vi "Main (1).vi"() -> ()   [LabVIEW 2013]
uses:
  <vilib>/myRIO/Common/Instrument Driver Framework/myRIO v1.0/UART/vis/myRIO v1.0 Close UART.vi
  <vilib>/functionblocks/Edge Detection/One Shot Rising with Input/One Shot Rising with Input.vi
  <vilib>/myRIO/Common/Instrument Driver Framework/Utilities/vis/FPGA Ref Manager.vi
  <vilib>/myRIO/Common/Instrument Driver Framework/myRIO v1.0/myRIO v1.0 Reset FPGA.vi
  <vilib>/functionblocks/FB Core/FB Core.xnode
  <vilib>/myRIO/Instrument Drivers/Utilities/Utilities.lvlib
  <vilib>/functionblocks/NI_FunctionBlock Libraries.lvlib
panel:
  in  "Tab Control 2":T1(tab)
  in  "Y Accel Rate (mm/s^2)":dbl
  in  "Y Decel Rate (mm/s^2)":dbl
  in  "Y Vmax (mm/s)":dbl
  in  "Y Vcreep (mm/s)":dbl
  in  "Y Creep  Distance (mm)":dbl
  in  "Y Overrun Distance (mm)":dbl
  in  "Y Target Coordinate Override (mm)":dbl min=0.0
  in  "Enable Y Coordinate Override":bool
  in  "Y-Axis Direction Request":bool
  in  "Y Axis Speed Override (mm/s)":dbl format="%#_13g"
  in  "Enable Y Axis Override":bool
  in  "Tab Control":T2(tab)
  in  "X Vmax (mm/s)":dbl
  in  "X Vcreep (mm/s)":dbl
  in  "X Overrun Distance (mm)":dbl
  in  "X Decel Rate (mm/s^2)":dbl
  in  "X Creep  Distance (mm)":dbl
  in  "X Accel Rate (mm/s^2)":dbl
  in  "X Target Coordinate (mm) 2":dbl min=0.0
  in  "Enable X Coordinate Override":bool
  in  "Enable X Axis Override":bool
  in  "X Axis Speed Override (mm/s)":dbl format="%#_13g"
  in  "X-Axis Direction Request":bool
  out "X Movement Timeout (s)":dbl caption="Elapsed Time (s)"
  out "X Target Coordinate (mm)":dbl min=0.0
  out "Y Target Coordinate (mm)":dbl min=0.0
  in  "Move to Specified Coordinate":bool
  in  "Calibrate Axes":bool
  out "Y Axis Frequency Command":dbl
  out "Y Axis Direction Command 3":bool
  out "Y_FiltSpeed(mm/s)":dbl
  out "Y_Dist_mm@(N)":dbl
  out "Y Axis":cluster{"Y":dbl[], "Y":dbl[]}[](graph)
  out "Y Speed Command (mm/s)":dbl
  out "Y Selected Speed Control Case":T3(ring)
  out "Active Y Axis Control Case":T4(ring)
  out "Active X Axis Control Case":T4(ring)
  out "X Speed Command (mm/s)":dbl
  out "X Selected Speed Control Case":T3(ring)
  out "X Axis":cluster{"Y":dbl[], "Y":dbl[]}[](graph)
  out "X_Dist_mm@(N)":dbl
  out "X_FiltSpeed(mm/s)":dbl
  out "X Axis Direction Command":bool
  out "X Axis Duty Command":dbl
  in  "Stop Button":bool
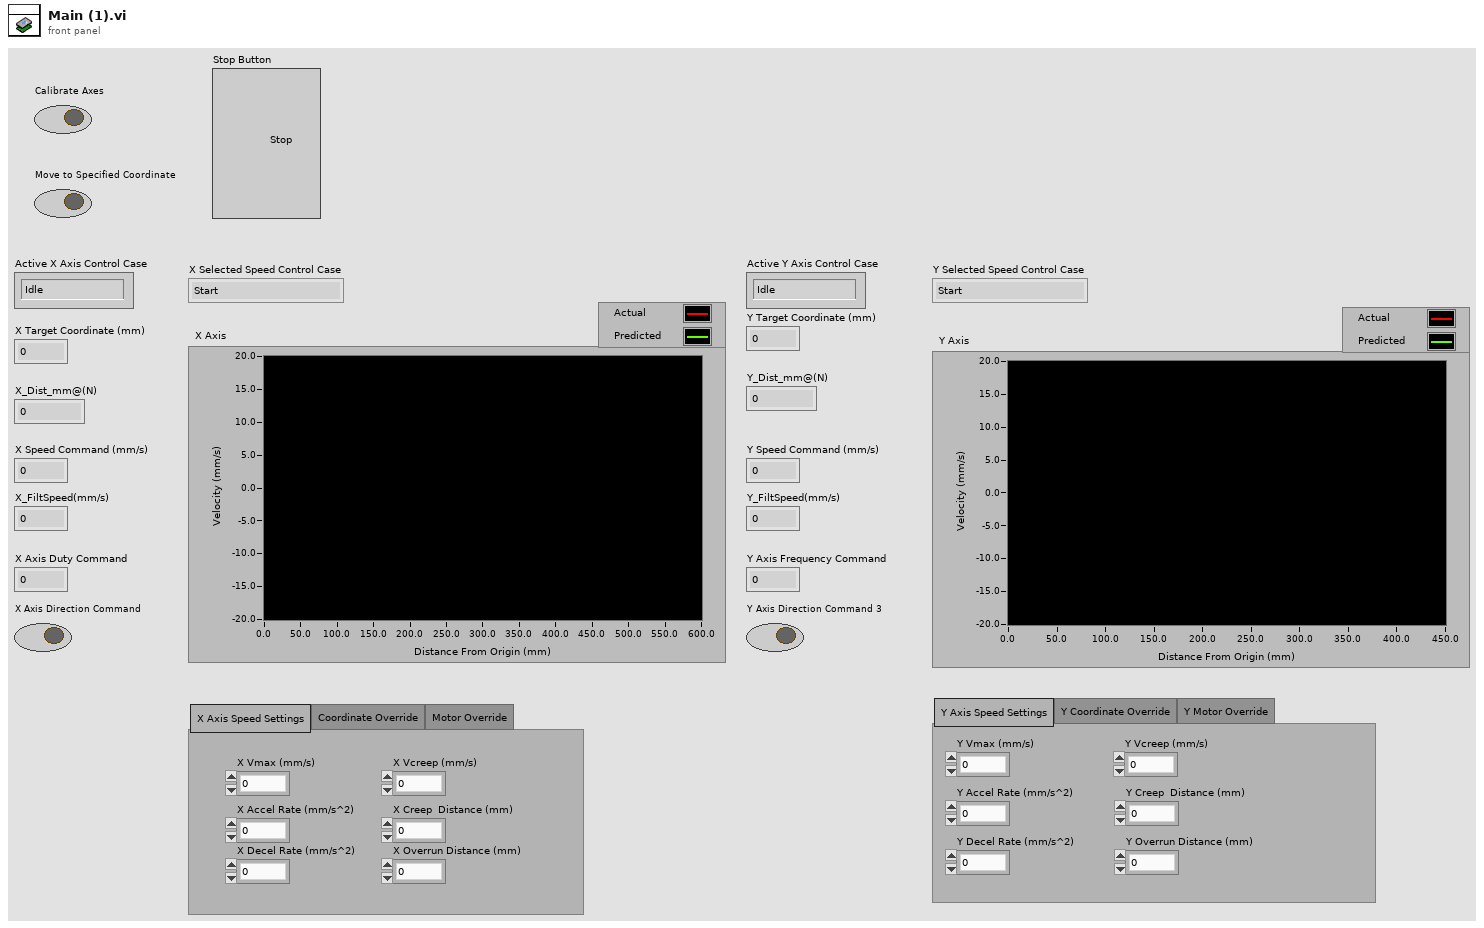
[diagram p1: front panel]
types:
  T1 = enum32{"Y Axis Speed Settings", "Y Coordinate Override", "Y Motor Override"}
  T2 = enum32{"X Axis Speed Settings", "Coordinate Override", "Motor Override"}
  T3 = enum16{"Start", "Accelerate", "Hold Vmax", "Decelerate", "Hold at Vcreep", "Stop"}
  T4 = enum16{"Idle", "PredictProfile", "Calibrate", "Home", "Go to Coordinate"}
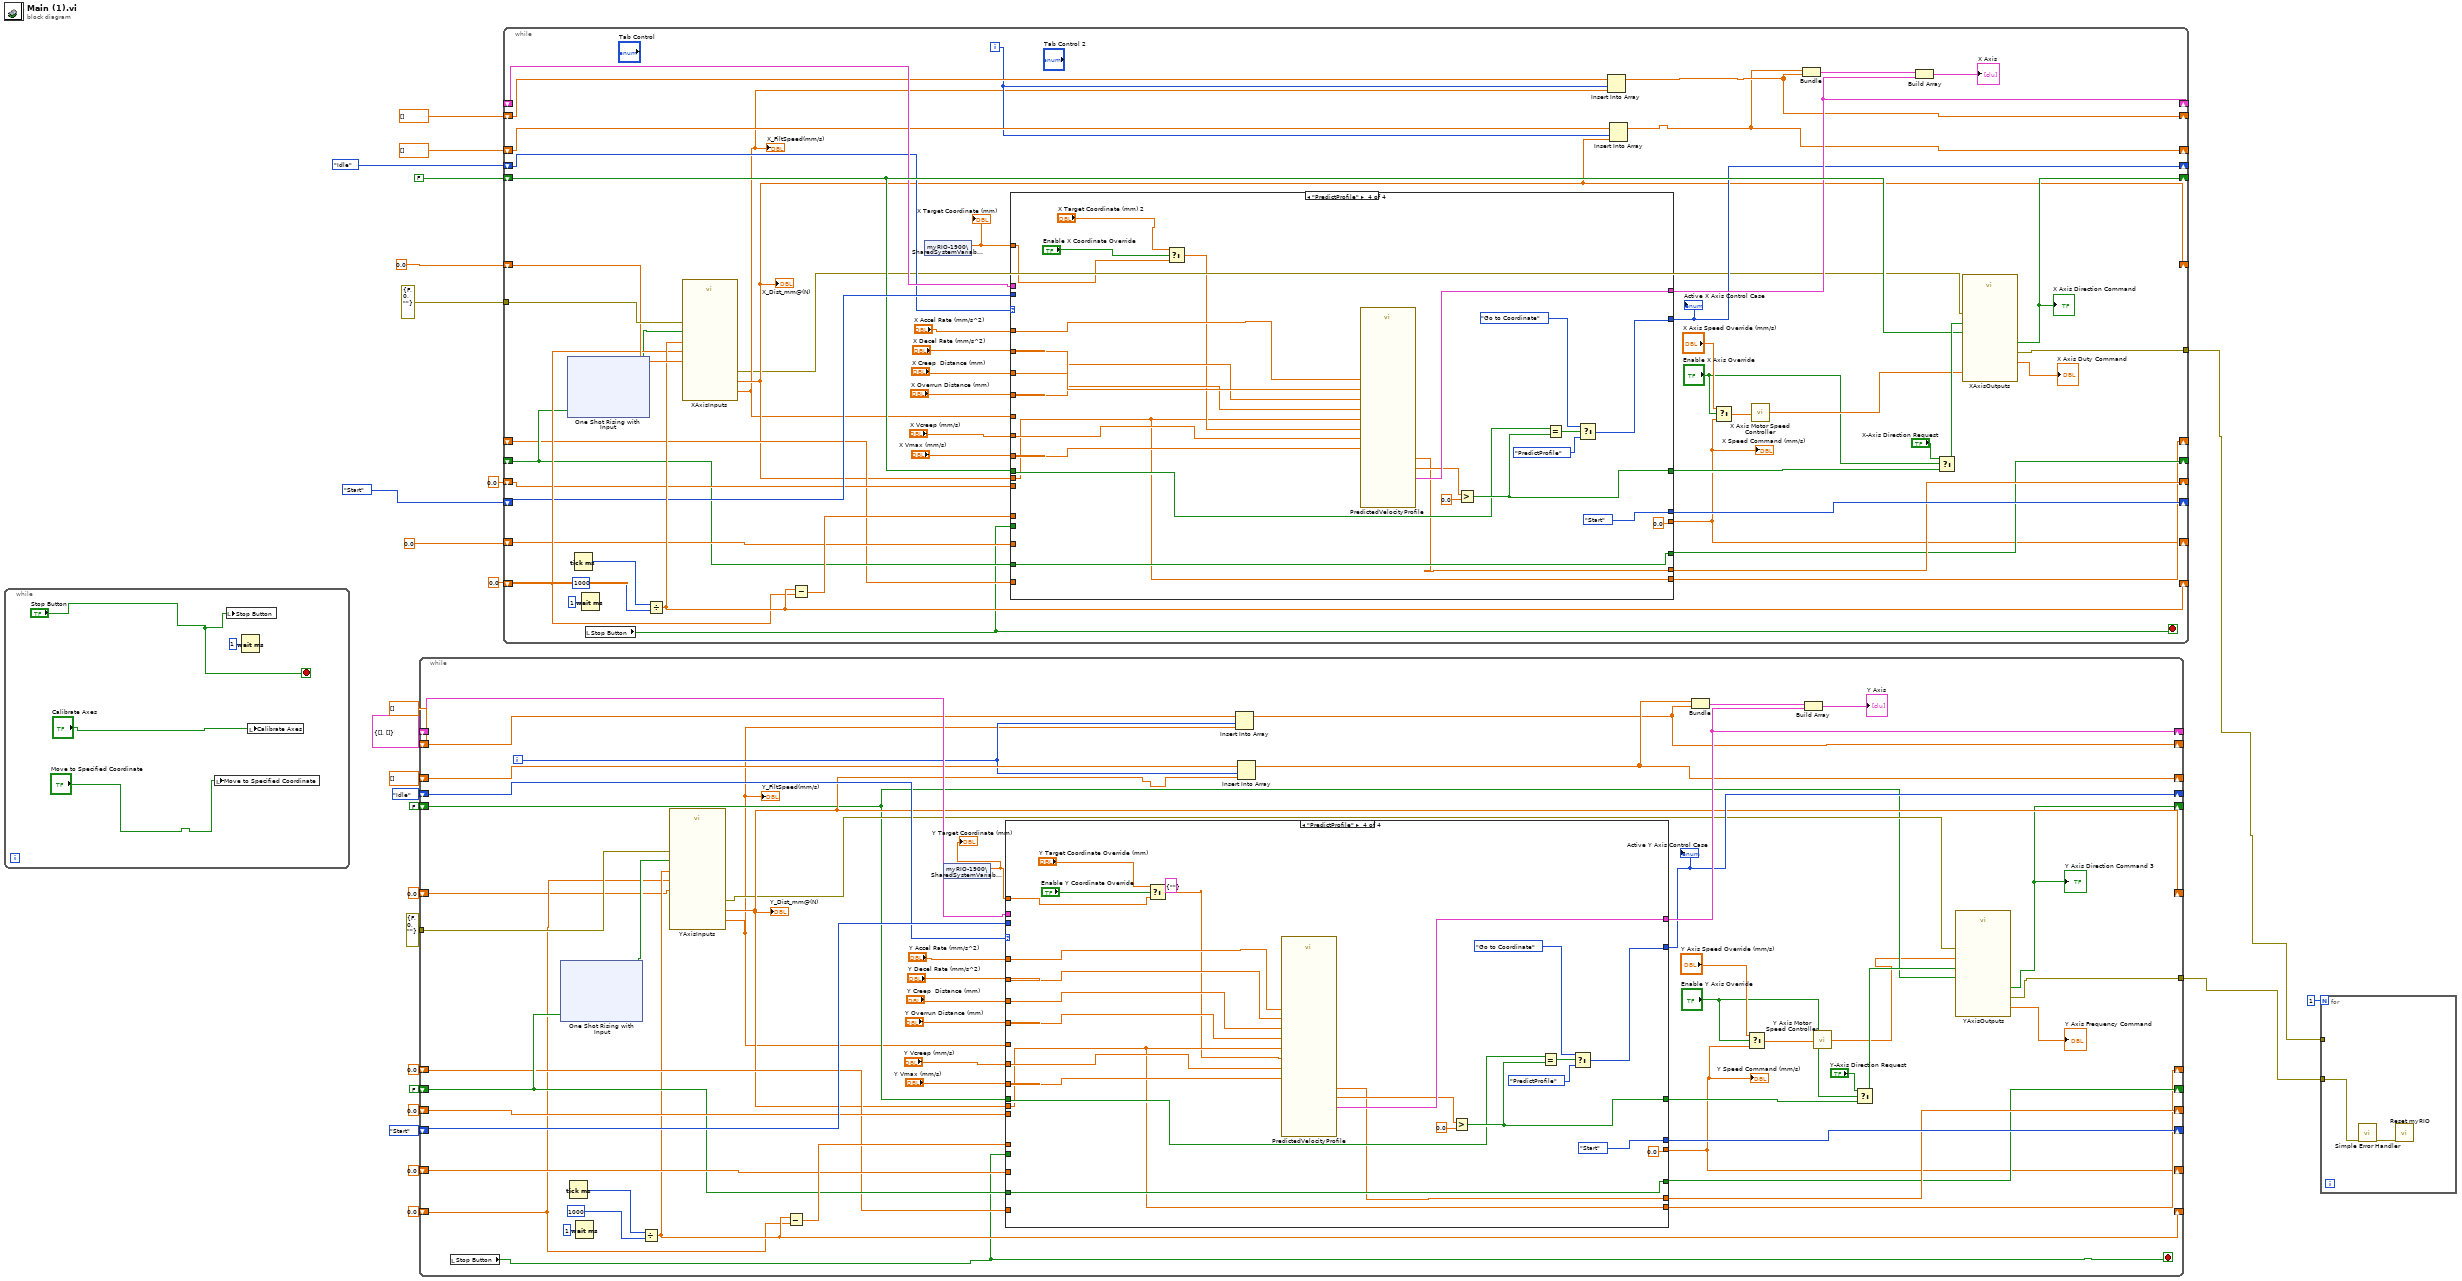
[diagram p0: block diagram]
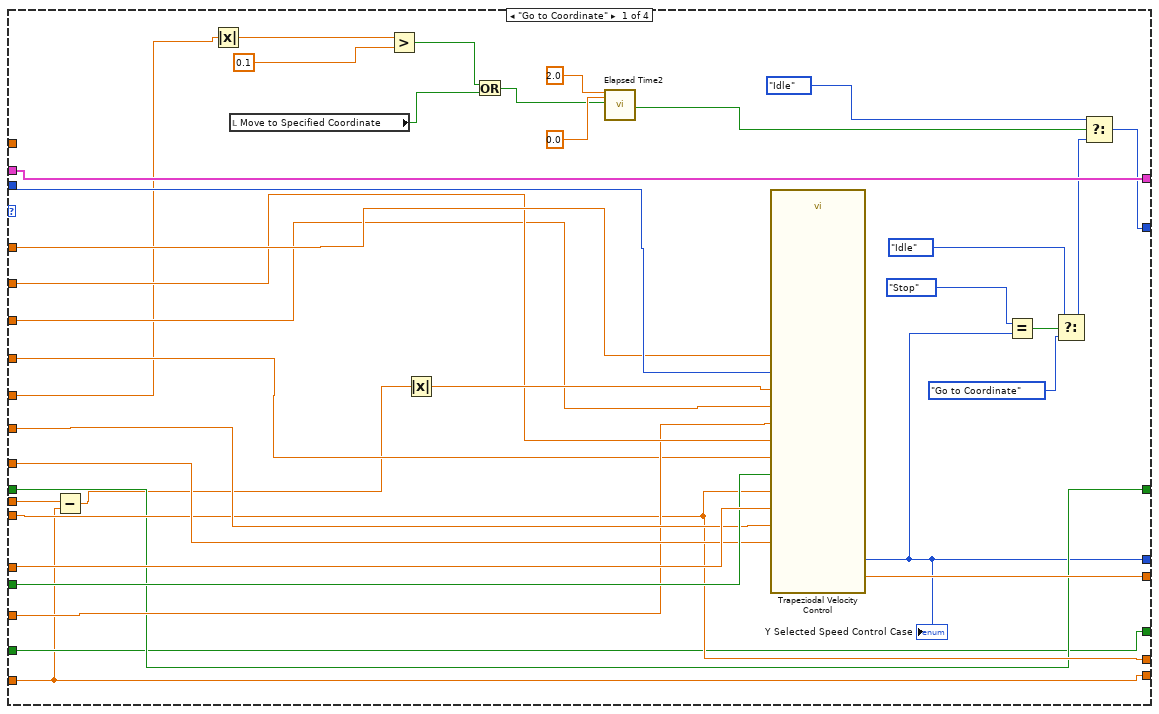
[diagram p2: hidden frame]
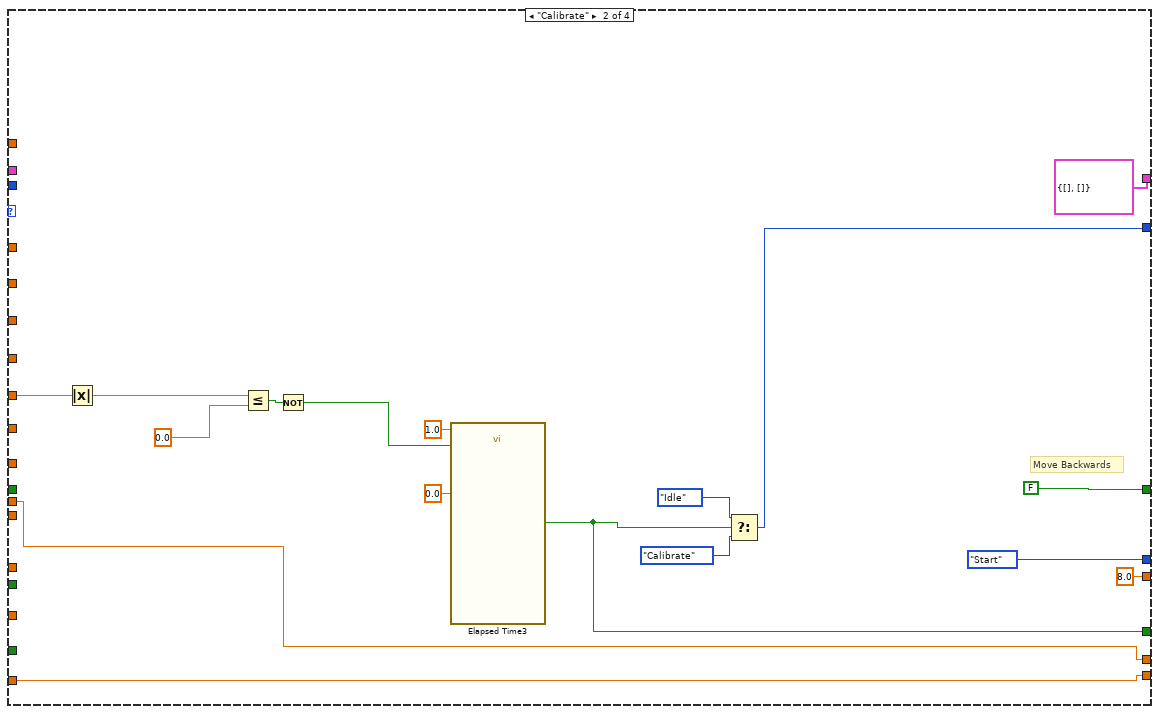
[diagram p3: hidden frame]
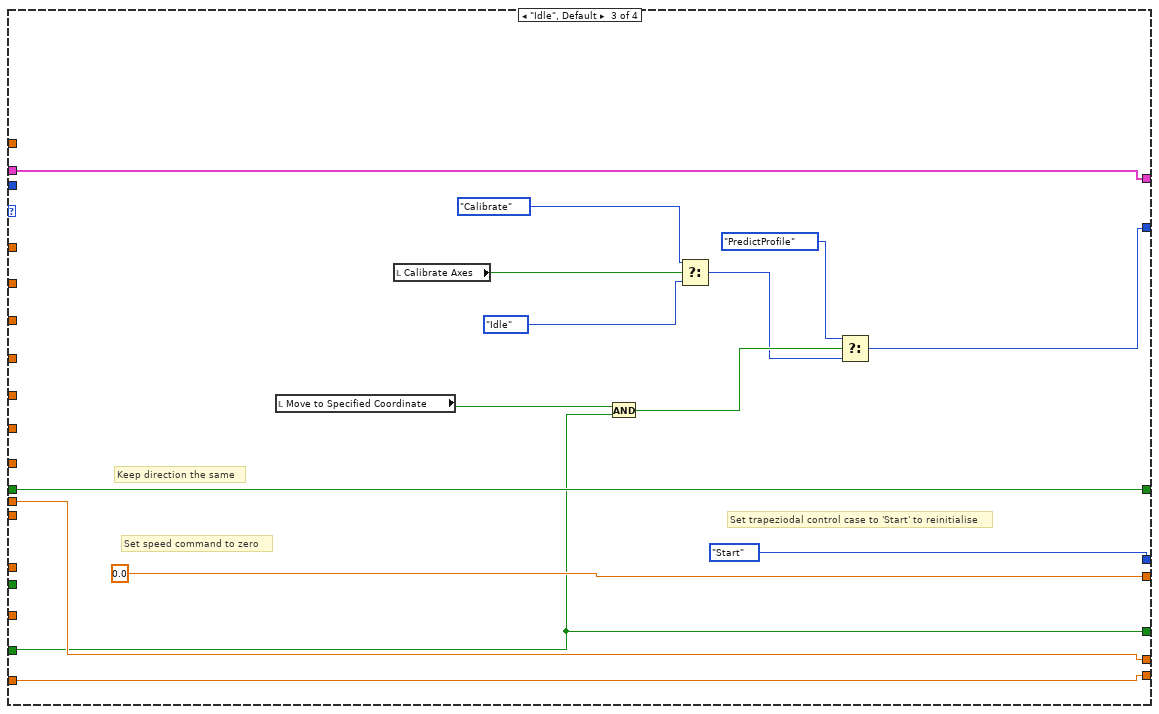
[diagram p4: hidden frame]
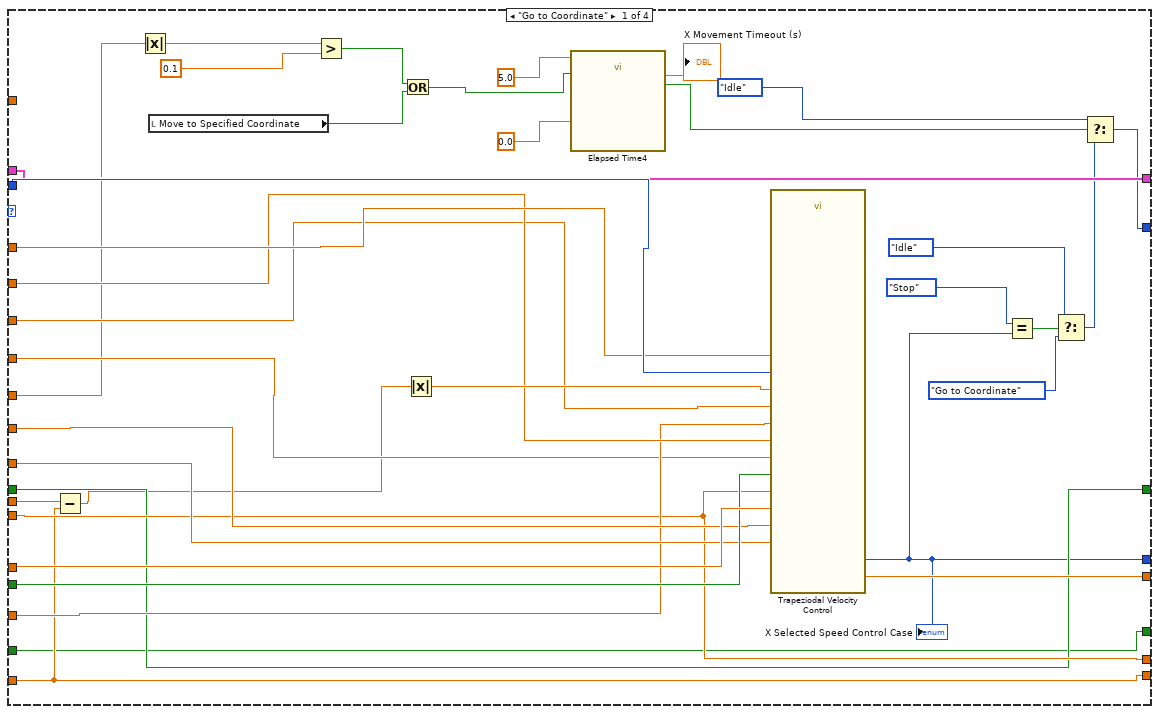
[diagram p5: hidden frame]
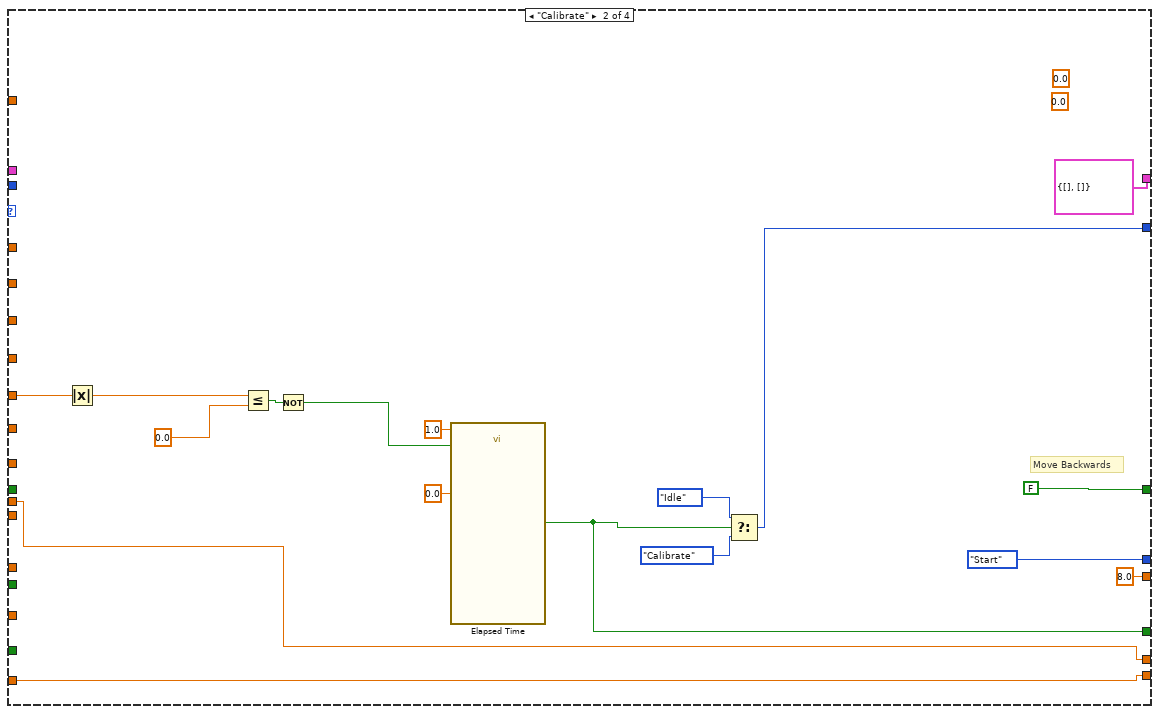
[diagram p6: hidden frame]
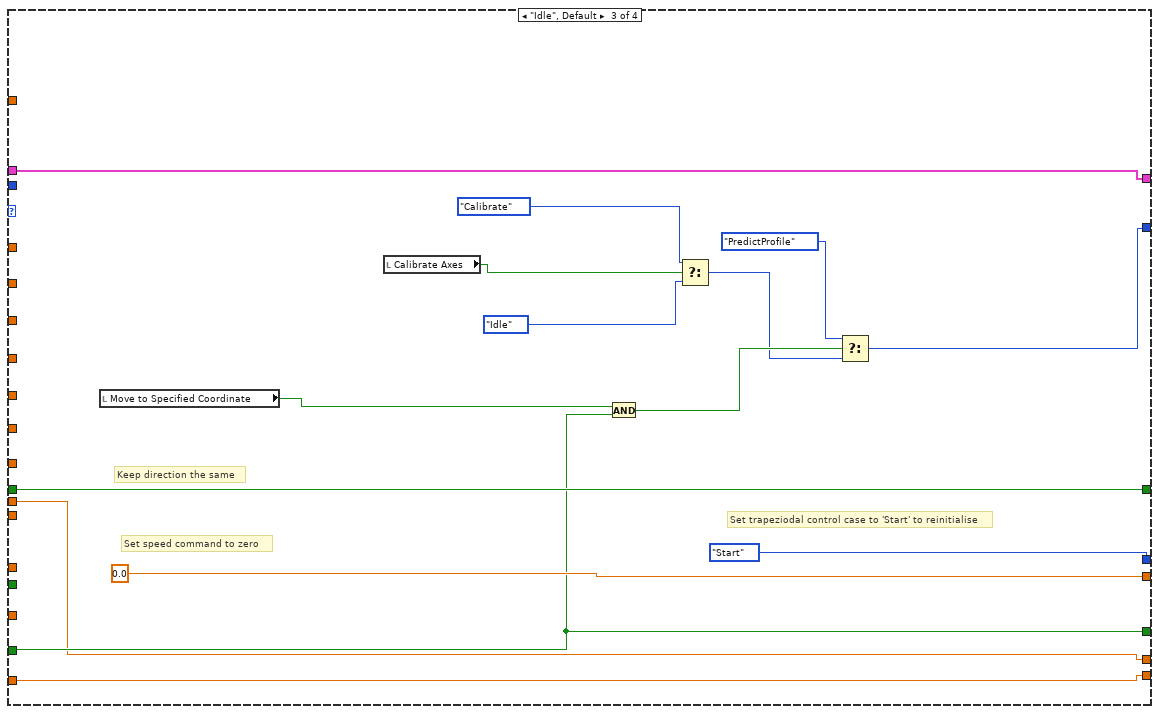
[diagram p7: hidden frame]
diagram:
  n1 = while {
    stop <- "Stop Button" stop-if-true
    n2 = local write "Move to Specified Coordinate"("Move to Specified Coordinate") -> ()
    n3 = local write "Stop Button"("Stop Button") -> ()
    n4 = Wait (ms)(milliseconds to wait=u32 1) -> ()  [unwired: 1 out]
    n5 = local write "Calibrate Axes"("Calibrate Axes") -> ()
  }
  n6 = while {
    shift-right: [w48] -> _
    shift-left: 0.0 -> [w46]
    tunnel: errorcluster {"status"=FALSE, "code"=0, "source"=""} ("error in (no error)") -> [w50]
    shift-right: [w41] -> _
    shift-left: FALSE ("Direction Command") -> [w42]
    tunnel: [w40] -> w1
    shift-right: [w47] -> _
    shift-left: 0.0 ("X_Dist_mm@(N)") -> [w45]
    shift-right: [w79] -> _
    shift-left: T3."Start" ("Selected Speed Control Case") -> [w74]
    shift-right: [w35] -> _
    shift-left: 0.0 ("Speed Command (mm/s)") -> [w66]
    shift-right: [w59] -> _
    shift-left: dbl[] [] -> [w57]
    shift-right: [w58] -> _
    shift-left: dbl[] [] -> [w54]
    shift-right: [w65] -> _
    shift-left: 0.0 ("Absolute Distance to Move (mm)") -> [w64]
    shift-right: [w63] -> _
    shift-left: cluster{dbl[], cdb[]} {[], []} ("PredictedVelocityProfile") -> [w62]
    shift-right: [w61] -> _
    shift-left: T4."Idle" ("Active X Axis Control Case") -> [w53]
    shift-right: [w60] -> _
    shift-left: FALSE ("Time has Elapsed") -> [w56]
    shift-right: [w52] -> _
    shift-left: 0.0 ("X_Dist_mm@(N)") -> [w51]
    i -> [w55]
    stop <- w32 stop-if-true
    n7 = local read "Stop Button"() -> (w32:bool)
    n8 = xnode "One Shot Rising with Input"("input"=w56) -> ("output"=w49:bool)  [unwired: 1 in, 1 out]
    n9 = Tick Count (ms)() -> (millisecond timer value=w81:u32)
    n10 = Wait (ms)(milliseconds to wait=u32 1) -> ()  [unwired: 1 out]
    n11 = Divide(x=w81, y=u32 1000) -> (x/y=w48:dbl)
    n12 = call "YAxisInputs.vi"("t_s"=w48, "error in (no error)"=w50, "t_s@(N-1)"=w46, "Reset Timer and Encoder Counts"=w49, "Y_Dist_mm@(N-1)"=w45) -> ("error out"=w44:errorcluster, "Y_Dist_mm@(N)"=w47:dbl, "Y_FiltSpeed(mm/s)"=w34:dbl)  [unwired: 4 in]
    "Y_FiltSpeed(mm/s)" <- w34
    "Y_Dist_mm@(N)" <- w47
    n13 = Subtract(x=w48, y=w46) -> (x-y=w78:dbl)
    n14 = shared-variable "myRIO-1900\\SharedSystemVariables.lvlib\\Puck Y"() -> (w39:dbl)  [unwired: 1 in, 1 out]
    "Y Target Coordinate (mm)" <- w39
    n15 = case shown="\"PredictProfile\"" w53 {
      tunnel: [w141 T3."Start" ("Selected Speed Control Case") T3."Start" ("Selected Speed Control Case") T3."Start" ("Selected Speed Control Case")] -> w79
      tunnel: w78 -> [w156 _ _ _]
      tunnel: w32 -> [w154 _ _ _]
      tunnel: [w153 8.0 ("Speed Command (mm/s)") 0.0 ("Speed Command (mm/s)") 0.0 ("Speed Command (mm/s)")] -> w35
      tunnel: w74 -> [w152 _ _ _]
      tunnel: [w143 FALSE ("Direction Command") w188 w200] -> w73
      tunnel: w42 -> [w143 _ w188 w199]
      tunnel: "Y Accel Rate (mm/s^2)" -> [w151 _ _ w212]
      tunnel: "Y Decel Rate (mm/s^2)" -> [w150 _ _ w211]
      tunnel: "Y Creep  Distance (mm)" -> [w149 _ _ w210]
      tunnel: "Y Overrun Distance (mm)" -> [w145 _ _ w209]
      tunnel: "Y Vcreep (mm/s)" -> [w148 _ _ w208]
      tunnel: "Y Vmax (mm/s)" -> [w147 _ _ w207]
      tunnel: w47 -> [w135 w173 w185 w193]
      tunnel: w66 -> [w146 _ _ _]
      tunnel: [w142 cluster{dbl[], cdb[]} {[], []} ("PredictedVelocityProfile") w178 w206] -> w63
      tunnel: [w144 w173 w185 w194] -> w65
      tunnel: w64 -> [w144 _ _ _]
      tunnel: w62 -> [w142 _ w178 _]
      tunnel: [w127 w166 w176 w196] -> w61
      tunnel: w34 -> [w123 w168 _ _]
      tunnel: [w136 w158 w179 w201] -> w60
      tunnel: w56 -> [w136 _ w179 w201]
      tunnel: [w133 w157 w177 w193] -> w52
      tunnel: w51 -> [w133 w157 w177 _]
      tunnel: w39 -> [_ _ _ w189]
      frame "Go to Coordinate" {
        n16 = Subtract(x=w135, y=w133) -> (x-y=w134:dbl)
        n17 = Absolute Value(x=w123) -> (abs(x)=w125:dbl)
        n18 = local read "Move to Specified Coordinate"() -> (w121:bool)
        n19 = Greater?(x=w125, y=0.1) -> (0:w124:bool)
        n20 = Absolute Value(x=w134) -> (abs(x)=w155:dbl)
        n21 = Or(x=w124, y=w121) -> (x .or. y?=w122:bool)
        n22 = call "Elapsed Time2"("Time Target (s)"=2.0, "Reset"=w122, "Set Start Time (s)"=0.0) -> ("Time has Elapsed"=w129:bool)  [unwired: 9 in, 7 out]
        n23 = call "Trapeziodal Velocity Control.vi"("Active Speed Control Case"=w152, "Vmax (mm/s)"=w147, "Accel Rate (mm/s^2)"=w151, "Decel Rate (mm/s^2) 2"=w150, "Current Speed (mm/s)"=w146, "Target Distance (mm)"=w144, "Actual Distance (mm)"=w155, "Creep  Distance (mm)"=w149, "Vcreep (mm/s)"=w148, "Overrun Distance (mm)"=w145, "Timestep (dt)"=w156, "stop or error"=w154) -> ("Selected Speed Control Case"=w141:T3, "Speed Command (mm/s)"=w153:dbl)  [unwired: 2 in]
        "Y Selected Speed Control Case" <- w141
        n24 = Equal?(x=T3."Stop" ("y"), y=w141) -> (x = y?=w139:bool)
        n25 = Select(t=T4."Idle" ("X Axis Control Case"), s=w139, f=T4."Go to Coordinate" ("X Axis Control Case")) -> (s? t:f=w128:T4)
        n26 = Select(t=T4."Idle" ("X Axis Control Case"), s=w129, f=w128) -> (s? t:f=w127:T4)
      }
      frame "Calibrate" {
        # "Move Backwards"
        n27 = Absolute Value(x=w168) -> (abs(x)=w163:dbl)
        n28 = Less Or Equal?(x=w163, y=0.0) -> (x <= y?=w162:bool)
        n29 = Not(x=w162) -> (.not. x?=w161:bool)
        n30 = call "Elapsed Time3"("Time Target (s)"=1.0, "Reset"=w161, "Set Start Time (s)"=0.0) -> ("Time has Elapsed"=w158:bool)  [unwired: 9 in, 7 out]
        n31 = Select(t=T4."Idle" ("X Axis Control Case"), s=w158, f=T4."Calibrate" ("X Axis Control Case")) -> (s? t:f=w166:T4)
      }
      frame "Idle", Default {
        # "Set trapeziodal control case to 'Start' to reinitialise"
        # "Set speed command to zero"
        # "Keep direction the same"
        n32 = local read "Move to Specified Coordinate"() -> (w174:bool)
        n33 = local read "Calibrate Axes"() -> (w175:bool)
        n34 = And(x=w174, y=w179) -> (x .and. y?=w182:bool)
        n35 = Select(t=T4."Calibrate" ("X Axis Control Case"), s=w175, f=T4."Idle" ("X Axis Control Case")) -> (s? t:f=w181:T4)
        n36 = Select(t=T4."PredictProfile" ("X Axis Control Case"), s=w182, f=w181) -> (s? t:f=w176:T4)
      }
      frame "PredictProfile" {
        (unwired) cluster{"source":string} {"source"=""} ("error in (no error)")
        n37 = Select(t="Y Target Coordinate Override (mm)", s="Enable Y Coordinate Override", f=w189) -> (s? t:f=w190:dbl)
        n38 = call "PredictedVelocityProfile.vi"("Start Coordinate (mm)"=w193, "V_Max_mm/s"=w207, "Accel_mm/s^2"=w212, "Target Coordinate (mm)"=w190, "S_Creep_mm"=w210, "S_Overrun_mm"=w209, "V_Creep_mm/s"=w208, "Decel_mm/s^2"=w211) -> ("Absolute Distance to Move (mm)"=w194:dbl, "Direction Request"=w204:dbl, "PredictedVelocityProfile"=w206:cluster{dbl[], cdb[]})  [unwired: 4 in, 1 out]
        n39 = Greater?(x=w204, y=0.0) -> (0:w200:bool)
        n40 = Equal?(x=w199, y=w200) -> (x = y?=w198:bool)
        n41 = Select(t=T4."Go to Coordinate" ("Active X Axis Control Case"), s=w198, f=T4."PredictProfile" ("Active X Axis Control Case")) -> (s? t:f=w196:T4)
      }
    }
    "Y Speed Command (mm/s)" <- w35
    "Active Y Axis Control Case" <- w61
    n42 = Insert Into Array(array=w54, index=w55, new element=w34) -> (w58:dbl[])
    n43 = Insert Into Array(array=w57, index=w55, new element=w47) -> (w59:dbl[])
    n44 = Bundle(w59, w58) -> (w76:cluster{dbl[], dbl[]})  [unwired: 1 in]
    n45 = Select(t="Y Axis Speed Override (mm/s)", s="Enable Y Axis Override", f=w35) -> (s? t:f=w36:dbl)
    n46 = Build Array(w76, w63) -> (→"Y Axis":cluster{dbl[], cdb[]}[])
    n47 = call "Y Axis Motor Speed Controller.vi"("Speed Command (mm/s)"=w36) -> ("PWM  Frequency Command (Hz)"=w33:dbl)
    n48 = Select(t="Y-Axis Direction Request", s="Enable Y Axis Override", f=w73) -> (s? t:f=w43:bool)
    n49 = call "YAxisOutputs.vi"("error in (no error)"=w44, "PWM  Frequency Command (Hz)"=w33, "YActiveDirectionCmd"=w42, "Y-Axis Direction Request"=w43) -> ("error out"=w40:errorcluster, "Limited Output"=→"Y Axis Frequency Command":dbl, "Direction Command"=w41:bool)  [unwired: 5 in]
    "Y Axis Direction Command 3" <- w41
  }
  n50 = while {
    shift-right: [w255] -> _
    shift-left: 0.0 -> [w254]
    tunnel: errorcluster {"status"=FALSE, "code"=0, "source"=""} ("error in (no error)") -> [w261]
    shift-right: [w259] -> _
    shift-left: FALSE ("Direction Command") -> [w247]
    tunnel: [w258] -> w18
    shift-right: [w224] -> _
    shift-left: 0.0 ("X_Dist_mm@(N)") -> [w257]
    shift-right: [w256] -> _
    shift-left: T3."Start" ("Selected Speed Control Case") -> [w249]
    shift-right: [w218] -> _
    shift-left: 0.0 ("Speed Command (mm/s)") -> [w240]
    shift-right: [w214] -> _
    shift-left: dbl[] [] -> [w233]
    shift-right: [w215] -> _
    shift-left: dbl[] [] -> [w231]
    shift-right: [w239] -> _
    shift-left: 0.0 ("Absolute Distance to Move (mm)") -> [w238]
    shift-right: [w237] -> _
    shift-left: _ -> [w236]
    shift-right: [w235] -> _
    shift-left: T4."Idle" ("X Axis Control Case") -> [w229]
    shift-right: [w234] -> _
    shift-left: _ -> [w232]
    shift-right: [w228] -> _
    shift-left: _ -> [w227]
    i -> [w223]
    stop <- w226 stop-if-true
    n51 = xnode "One Shot Rising with Input"("input"=w232) -> ("output"=w230:bool)  [unwired: 1 in, 1 out]
    n52 = Tick Count (ms)() -> (millisecond timer value=w263:u32)
    n53 = Wait (ms)(milliseconds to wait=u32 1) -> ()  [unwired: 1 out]
    n54 = local read "Stop Button"() -> (w226:bool)
    n55 = Divide(x=w263, y=u32 1000) -> (x/y=w255:dbl)
    n56 = call "XAxisInputs.vi"("t_s"=w255, "error in (no error)"=w261, "t_s@(N-1)"=w254, "Reset Timer and Encoder Counts"=w230, "X_Dist_mm@(N-1)"=w257) -> ("error out"=w216:errorcluster, "X_Dist_mm@(N)"=w224:dbl, "X_FiltSpeed(mm/s)"=w217:dbl)  [unwired: 4 in]
    "X_FiltSpeed(mm/s)" <- w217
    "X_Dist_mm@(N)" <- w224
    n57 = Subtract(x=w255, y=w254) -> (x-y=w253:dbl)
    n58 = shared-variable "myRIO-1900\\SharedSystemVariables.lvlib\\Puck X"() -> (w225:dbl)  [unwired: 1 in, 1 out]
    "X Target Coordinate (mm)" <- w225
    n59 = case shown="\"PredictProfile\"" w229 {
      tunnel: [w324 T3."Start" ("Selected Speed Control Case") T3."Start" ("Selected Speed Control Case") T3."Start" ("Selected Speed Control Case")] -> w256
      tunnel: w253 -> [w339 _ _ _]
      tunnel: w226 -> [w337 _ _ _]
      tunnel: [w336 8.0 ("Speed Command (mm/s)") 0.0 ("Speed Command (mm/s)") 0.0 ("Speed Command (mm/s)")] -> w218
      tunnel: w249 -> [w335 _ _ _]
      tunnel: [w326 FALSE ("Direction Command") w371 w383] -> w248
      tunnel: w247 -> [w326 _ w371 w382]
      tunnel: "X Accel Rate (mm/s^2)" -> [w334 _ _ w395]
      tunnel: "X Decel Rate (mm/s^2)" -> [w333 _ _ w394]
      tunnel: "X Creep  Distance (mm)" -> [w332 _ _ w393]
      tunnel: "X Overrun Distance (mm)" -> [w328 _ _ w392]
      tunnel: "X Vcreep (mm/s)" -> [w331 _ _ w391]
      tunnel: "X Vmax (mm/s)" -> [w330 _ _ w390]
      tunnel: w224 -> [w317 w356 w358 w372]
      tunnel: w240 -> [w329 _ _ _]
      tunnel: [w325 cluster{dbl[], cdb[]} {[], []} ("PredictedVelocityProfile") w363 w389] -> w237
      tunnel: [w327 w356 w358 w377] -> w239
      tunnel: w238 -> [w327 _ _ _]
      tunnel: w236 -> [w325 _ w363 _]
      tunnel: [w309 w349 w361 w379] -> w235
      tunnel: w217 -> [w308 w351 _ _]
      tunnel: [w306 w341 w359 w384] -> w234
      tunnel: w232 -> [w306 _ w359 w384]
      tunnel: [w318 w340 w362 w372] -> w228
      tunnel: w227 -> [w318 w340 w362 _]
      tunnel: w225 -> [_ _ _ w373]
      frame "Go to Coordinate" {
        n60 = Subtract(x=w317, y=w318) -> (x-y=w319:dbl)
        n61 = Absolute Value(x=w308) -> (abs(x)=w314:dbl)
        n62 = local read "Move to Specified Coordinate"() -> (w303:bool)
        n63 = Greater?(x=w314, y=0.1) -> (0:w304:bool)
        n64 = Or(x=w304, y=w303) -> (x .or. y?=w305:bool)
        n65 = Absolute Value(x=w319) -> (abs(x)=w338:dbl)
        n66 = call "Elapsed Time4"("Time Target (s)"=5.0, "Reset"=w305, "Set Start Time (s)"=0.0) -> ("Elapsed Time (s)"=→"X Movement Timeout (s)":dbl, "Time has Elapsed"=w311:bool)  [unwired: 9 in, 6 out]
        n67 = call "Trapeziodal Velocity Control.vi"("Active Speed Control Case"=w335, "Vmax (mm/s)"=w330, "Accel Rate (mm/s^2)"=w334, "Decel Rate (mm/s^2) 2"=w333, "Current Speed (mm/s)"=w329, "Target Distance (mm)"=w327, "Actual Distance (mm)"=w338, "Creep  Distance (mm)"=w332, "Vcreep (mm/s)"=w331, "Overrun Distance (mm)"=w328, "Timestep (dt)"=w339, "stop or error"=w337) -> ("Selected Speed Control Case"=w324:T3, "Speed Command (mm/s)"=w336:dbl)  [unwired: 2 in]
        "X Selected Speed Control Case" <- w324
        n68 = Equal?(x=T3."Stop" ("y"), y=w324) -> (x = y?=w322:bool)
        n69 = Select(t=T4."Idle" ("X Axis Control Case"), s=w322, f=T4."Go to Coordinate" ("X Axis Control Case")) -> (s? t:f=w310:T4)
        n70 = Select(t=T4."Idle" ("X Axis Control Case"), s=w311, f=w310) -> (s? t:f=w309:T4)
      }
      frame "Calibrate" {
        (unwired) 0.0 ("f")
        (unwired) 0.0 ("f")
        # "Move Backwards"
        n71 = Absolute Value(x=w351) -> (abs(x)=w346:dbl)
        n72 = Less Or Equal?(x=w346, y=0.0) -> (x <= y?=w345:bool)
        n73 = Not(x=w345) -> (.not. x?=w344:bool)
        n74 = call "Elapsed Time"("Time Target (s)"=1.0, "Reset"=w344, "Set Start Time (s)"=0.0) -> ("Time has Elapsed"=w341:bool)  [unwired: 9 in, 7 out]
        n75 = Select(t=T4."Idle" ("X Axis Control Case"), s=w341, f=T4."Calibrate" ("X Axis Control Case")) -> (s? t:f=w349:T4)
      }
      frame "Idle", Default {
        # "Set trapeziodal control case to 'Start' to reinitialise"
        # "Set speed command to zero"
        # "Keep direction the same"
        n76 = local read "Move to Specified Coordinate"() -> (w357:bool)
        n77 = local read "Calibrate Axes"() -> (w360:bool)
        n78 = And(x=w357, y=w359) -> (x .and. y?=w366:bool)
        n79 = Select(t=T4."Calibrate" ("X Axis Control Case"), s=w360, f=T4."Idle" ("X Axis Control Case")) -> (s? t:f=w365:T4)
        n80 = Select(t=T4."PredictProfile" ("X Axis Control Case"), s=w366, f=w365) -> (s? t:f=w361:T4)
      }
      frame "PredictProfile" {
        n81 = Select(t="X Target Coordinate (mm) 2", s="Enable X Coordinate Override", f=w373) -> (s? t:f=w375:dbl)
        n82 = call "PredictedVelocityProfile.vi"("Start Coordinate (mm)"=w372, "V_Max_mm/s"=w390, "Accel_mm/s^2"=w395, "Target Coordinate (mm)"=w375, "S_Creep_mm"=w393, "S_Overrun_mm"=w392, "V_Creep_mm/s"=w391, "Decel_mm/s^2"=w394) -> ("Absolute Distance to Move (mm)"=w377:dbl, "Direction Request"=w387:dbl, "PredictedVelocityProfile"=w389:cluster{dbl[], cdb[]})  [unwired: 4 in, 1 out]
        n83 = Greater?(x=w387, y=0.0) -> (0:w383:bool)
        n84 = Equal?(x=w382, y=w383) -> (x = y?=w381:bool)
        n85 = Select(t=T4."Go to Coordinate" ("Active X Axis Control Case"), s=w381, f=T4."PredictProfile" ("Active X Axis Control Case")) -> (s? t:f=w379:T4)
      }
    }
    "X Speed Command (mm/s)" <- w218
    "Active X Axis Control Case" <- w235
    n86 = Insert Into Array(array=w231, index=w223, new element=w217) -> (w215:dbl[])
    n87 = Insert Into Array(array=w233, index=w223, new element=w224) -> (w214:dbl[])
    n88 = Select(t="X Axis Speed Override (mm/s)", s="Enable X Axis Override", f=w218) -> (s? t:f=w221:dbl)
    n89 = call "X Axis Motor Speed Controller.vi"("Speed Command (mm/s)"=w221) -> ("PWM  Duty Cycle Command (Hz)"=w222:dbl)
    n90 = Bundle(w214, w215) -> (w213:cluster{dbl[], dbl[]})  [unwired: 1 in]
    n91 = Build Array(w213, w237) -> (→"X Axis":cluster{dbl[], cdb[]}[])
    n92 = Select(t="X-Axis Direction Request", s="Enable X Axis Override", f=w248) -> (s? t:f=w251:bool)
    n93 = call "XAxisOutputs.vi"("error in (no error)"=w216, "PWM  Duty Cycle Command"=w222, "XActiveDirectionCmd"=w247, "X-Axis Direction Request"=w251) -> ("error out"=w258:errorcluster, "Limited Output"=→"X Axis Duty Command":dbl, "Direction Command"=w259:bool)  [unwired: 5 in]
    "X Axis Direction Command" <- w259
  }
  n94 = for {
    N: 1 -> [_]
    tunnel: w1 -> [w396]
    tunnel: w18 -> [_]
    n95 = call <vilib>:"Simple Error Handler.vi"("error in (no error)"=w396) -> ("error out"=w397:errorcluster)  [unwired: 4 in, 4 out]
    n96 = call <vilib>:"Reset myRIO.vi"("error in (no error)"=w397) -> ()  [unwired: 10 in, 1 out]
  }
